vi "Configure Slew Rate.vi"(8 "error in (no error)":errorcluster, 9 "Negative Slew Rate (1)":dbl=1.0 min=0.0001 max=2.5 step=0.001 format="%#.4f", 10 "Positive Slew Rate (1)":dbl=1.0 min=0.0001 max=2.5 step=0.001 format="%#.4f", 11 "VISA resource name":refnum<visa-resource-name>) -> (0 "error out":errorcluster, 3 "VISA resource name out":refnum<visa-resource-name>)   [LabVIEW 2018, in "BK Precision 8600 Series.lvlib"]
doc: "Configures the slew rate for constant current (CC) operation. Not available in all other operation modes."
uses:
  <instrlib>/BK Precision 8600 Series/BK Precision 8600 Series.lvlib
panel:
  # "A/us"
  # "A/us"
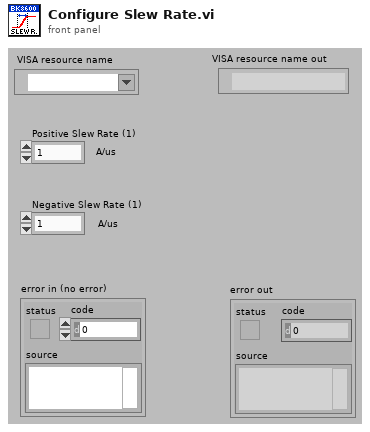
[diagram p1: front panel]
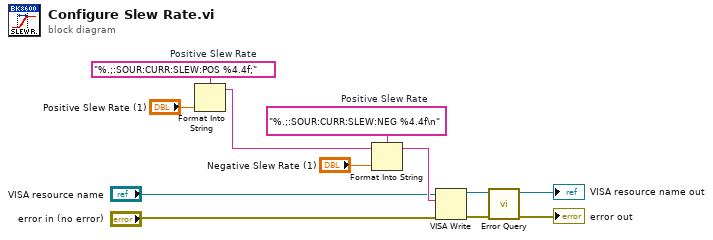
[diagram p0: block diagram]
diagram:
  w5 = "%.;:SOUR:CURR:SLEW:NEG %4.4f\n"  # Positive Slew Rate
  w8 = "%.;:SOUR:CURR:SLEW:POS %4.4f;"  # Positive Slew Rate
  n1 = Format Into String(format string=w8, "Positive Slew Rate (1)") -> (resulting string=w3:string)  [unwired: 2 in, 1 out]
  n2 = Format Into String(format string=w5, initial string=w3, "Negative Slew Rate (1)") -> (resulting string=w4:string)  [unwired: 1 in, 1 out]
  n3 = VISA Write(VISA resource name="VISA resource name", write buffer=w4, error in (no error)="error in (no error)") -> (VISA resource name out=w9:refnum<visa-resource-name>, error out=w10:errorcluster)  [unwired: 1 out]
  n4 = call <instrlib>:"Error Query.vi"("error in (no error)"=w10, "VISA resource name"=w9) -> ("error out"=→"error out":errorcluster, "VISA resource name out"=→"VISA resource name out":refnum<visa-resource-name>)  [unwired: 6 in, 2 out]
